vi "subDrawScaledCircle.vi"(0 "picture in":picture, 1 "Radius":i16, 2 "fill?(F)":bool, 5 "X":sgl, 7 "Y":sgl, 9 "Display Size":cluster{"Width":sgl, "Height":sgl}, 12 "color(black)":u32(colorbox)) -> (4 "picture out":picture)   [LabVIEW 2010]
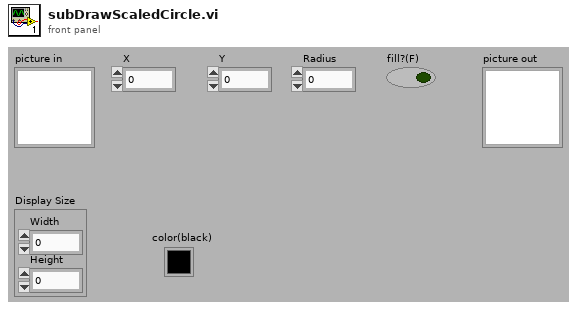
[diagram p1: front panel]
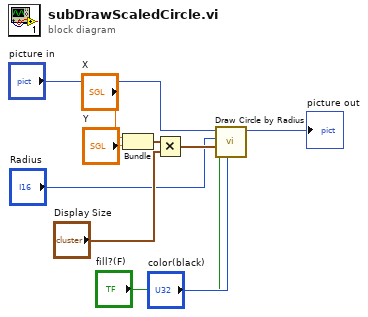
[diagram p0: block diagram]
diagram:
  n1 = Bundle("X"="X", "Y"="Y") -> (w6:cluster{"X":sgl, "Y":sgl})  [unwired: 1 out]
  n2 = Multiply(x=w6, y="Display Size") -> (x*y=w8:cluster{sgl, sgl})
  n3 = call <vilib>:"Draw Circle by Radius.vi"("color(black)"="color(black)", "fill?(F)"="fill?(F)", "pixel center"=w8, "radius"="Radius", "picture"="picture in") -> ("new picture"=→"picture out":picture)  [unwired: 3 in, 3 out]
